vi "INS_civitanavi_write_PXI_subvi.vi"(4 "Send":bool, 8 "NavOn":bool, 9 "Init":bool, 11 "Cluster":T1={"Offset Roll"=0.726926, "Offset Pitch"=-0.17842, "Offset Heading"=0.0310803, "Azimuth"=0.0, "Latitude "=-23.213156, "Longitude"=-45.860622, "Height"=622.367, "LP_Vel_Z-North"=0.0, "LP_Vel_Y-East"=0.0, "LP_Vel_X-Up"=0.0}) -> (3 "string out":string)   [LabVIEW 2017]
panel:
  in  "Fact Reserved":bool
  in  "Download":bool
  in  "Fact Config":bool
  out "Half Second":bool[][](array[boolean])=[[FALSE, FALSE, FALSE, FALSE, FALSE, FALSE, FALSE, FALSE, FALSE, FALSE], [FALSE, FALSE, TRUE, TRUE, TRUE, TRUE, TRUE, FALSE, FALSE, FALSE], [FALSE, TRUE, FALSE, FALSE, FALSE, FALSE, FALSE, TRUE, FALSE, FALSE], [FALSE, TRUE, FALSE, FALSE, FALSE, FALSE, FALSE, TRUE, FALSE, FALSE], [FALSE, TRUE, FALSE, FALSE, FALSE, FALSE, FALSE, TRUE, FALSE, FALSE], [FALSE, TRUE, FALSE, FALSE, FALSE, FALSE, FALSE, TRUE, FALSE, FALSE], [FALSE, TRUE, FALSE, FALSE, FALSE, FALSE, FALSE, TRUE, FALSE, FALSE], [FALSE, TRUE, FALSE, FALSE, FALSE, FALSE, FALSE, TRUE, FALSE, FALSE], [FALSE, FALSE, TRUE, TRUE, TRUE, TRUE, TRUE, FALSE, FALSE, FALSE], [FALSE, FALSE, FALSE, FALSE, FALSE, FALSE, FALSE, FALSE, FALSE, FALSE]]
  out "Min 1":bool[][](array[boolean])=[[FALSE, FALSE, FALSE, FALSE, FALSE, FALSE, FALSE, FALSE, FALSE, FALSE], [FALSE, FALSE, TRUE, TRUE, TRUE, TRUE, TRUE, FALSE, FALSE, FALSE], [FALSE, TRUE, FALSE, FALSE, FALSE, FALSE, FALSE, TRUE, FALSE, FALSE], [FALSE, TRUE, FALSE, FALSE, FALSE, FALSE, FALSE, TRUE, FALSE, FALSE], [FALSE, TRUE, FALSE, FALSE, FALSE, FALSE, FALSE, TRUE, FALSE, FALSE], [FALSE, TRUE, FALSE, FALSE, FALSE, FALSE, FALSE, TRUE, FALSE, FALSE], [FALSE, TRUE, FALSE, FALSE, FALSE, FALSE, FALSE, TRUE, FALSE, FALSE], [FALSE, TRUE, FALSE, FALSE, FALSE, FALSE, FALSE, TRUE, FALSE, FALSE], [FALSE, FALSE, TRUE, TRUE, TRUE, TRUE, TRUE, FALSE, FALSE, FALSE], [FALSE, FALSE, FALSE, FALSE, FALSE, FALSE, FALSE, FALSE, FALSE, FALSE]]
  out "Min 0":bool[][](array[boolean])=[[FALSE, FALSE, FALSE, FALSE, FALSE, FALSE, FALSE, FALSE, FALSE, FALSE], [FALSE, FALSE, TRUE, TRUE, TRUE, TRUE, TRUE, FALSE, FALSE, FALSE], [FALSE, TRUE, FALSE, FALSE, FALSE, FALSE, FALSE, TRUE, FALSE, FALSE], [FALSE, TRUE, FALSE, FALSE, FALSE, FALSE, FALSE, TRUE, FALSE, FALSE], [FALSE, TRUE, FALSE, FALSE, FALSE, FALSE, FALSE, TRUE, FALSE, FALSE], [FALSE, TRUE, FALSE, FALSE, FALSE, FALSE, FALSE, TRUE, FALSE, FALSE], [FALSE, TRUE, FALSE, FALSE, FALSE, FALSE, FALSE, TRUE, FALSE, FALSE], [FALSE, TRUE, FALSE, FALSE, FALSE, FALSE, FALSE, TRUE, FALSE, FALSE], [FALSE, FALSE, TRUE, TRUE, TRUE, TRUE, TRUE, FALSE, FALSE, FALSE], [FALSE, FALSE, FALSE, FALSE, FALSE, FALSE, FALSE, FALSE, FALSE, FALSE]]
  out "Hour 1":bool[][](array[boolean])=[[FALSE, FALSE, FALSE, FALSE, FALSE, FALSE, FALSE, FALSE, FALSE, FALSE], [FALSE, FALSE, TRUE, TRUE, TRUE, TRUE, TRUE, FALSE, FALSE, FALSE], [FALSE, TRUE, FALSE, FALSE, FALSE, FALSE, FALSE, TRUE, FALSE, FALSE], [FALSE, TRUE, FALSE, FALSE, FALSE, FALSE, FALSE, TRUE, FALSE, FALSE], [FALSE, TRUE, FALSE, FALSE, FALSE, FALSE, FALSE, TRUE, FALSE, FALSE], [FALSE, TRUE, FALSE, FALSE, FALSE, FALSE, FALSE, TRUE, FALSE, FALSE], [FALSE, TRUE, FALSE, FALSE, FALSE, FALSE, FALSE, TRUE, FALSE, FALSE], [FALSE, TRUE, FALSE, FALSE, FALSE, FALSE, FALSE, TRUE, FALSE, FALSE], [FALSE, FALSE, TRUE, TRUE, TRUE, TRUE, TRUE, FALSE, FALSE, FALSE], [FALSE, FALSE, FALSE, FALSE, FALSE, FALSE, FALSE, FALSE, FALSE, FALSE]]
  out "Hour 0":bool[][](array[boolean])=[[FALSE, FALSE, FALSE, FALSE, FALSE, FALSE, FALSE, FALSE, FALSE, FALSE], [FALSE, FALSE, TRUE, TRUE, TRUE, TRUE, TRUE, FALSE, FALSE, FALSE], [FALSE, TRUE, FALSE, FALSE, FALSE, FALSE, FALSE, TRUE, FALSE, FALSE], [FALSE, TRUE, FALSE, FALSE, FALSE, FALSE, FALSE, TRUE, FALSE, FALSE], [FALSE, TRUE, FALSE, FALSE, FALSE, FALSE, FALSE, TRUE, FALSE, FALSE], [FALSE, TRUE, FALSE, FALSE, FALSE, FALSE, FALSE, TRUE, FALSE, FALSE], [FALSE, TRUE, FALSE, FALSE, FALSE, FALSE, FALSE, TRUE, FALSE, FALSE], [FALSE, TRUE, FALSE, FALSE, FALSE, FALSE, FALSE, TRUE, FALSE, FALSE], [FALSE, FALSE, TRUE, TRUE, TRUE, TRUE, TRUE, FALSE, FALSE, FALSE], [FALSE, FALSE, FALSE, FALSE, FALSE, FALSE, FALSE, FALSE, FALSE, FALSE]]
  out "string in":string
  out "DV_Word":bool[](array[boolean])
  out "B_55":u8 format="%x"
  out "B_54":u8 format="%x"
  out "String":string
  # "B#55 (Configuration and Command Mode)"
  # "0x35"
  # "roll 0.229593"
  # "0xBD"
  # "pitch 0.442368"
  # "0XFA"
  # "yaw 0.00104293"
  # "0XEE"
  # "0XAB"
  # "0.128098 LP_Y-East"
  # "Não deixar os botões selecionados"
  # "0.467339 LP_Z-North"
  # "B#54 (Data Validity Word)"
  # "1= Installation Offset input valid data\n1= Launch Azimuth geodetic orientation, position, (lat, long, height) valid \n1= Velocity input valid data \nRFU\nRFU\nRFU\n 7,6     00= \"Init Cmd\" (Configuration parameters setting)\n           10= \"NAV_On\"\n           01= Reserved\n           11= Enter Configuration Mode"
  # "0\n1\n2\n3\n4\n5\n6\n7"
  # "Atualizar os valores das variaveis e pulsar o botão send"
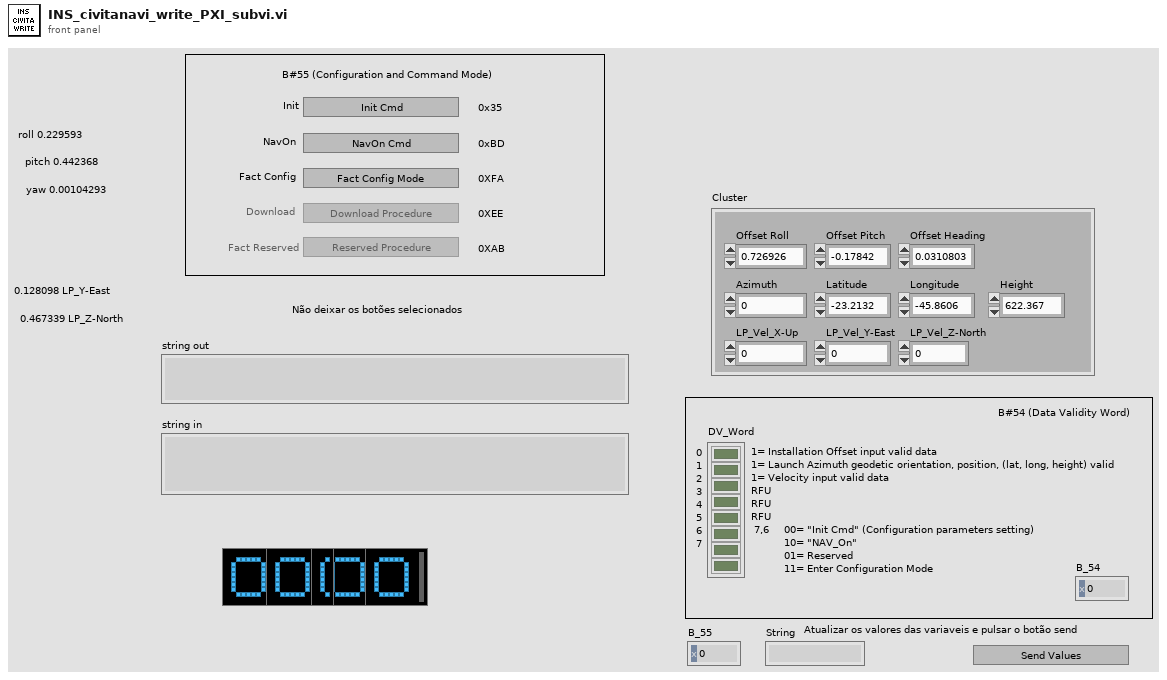
[diagram p1: front panel]
types:
  T1 = cluster{"Offset Roll":sgl, "Offset Pitch":sgl, "Offset Heading":sgl, "Azimuth":sgl, "Latitude ":sgl, "Longitude":sgl, "Height":sgl, "LP_Vel_Z-North":sgl, "LP_Vel_Y-East":sgl, "LP_Vel_X-Up":sgl}
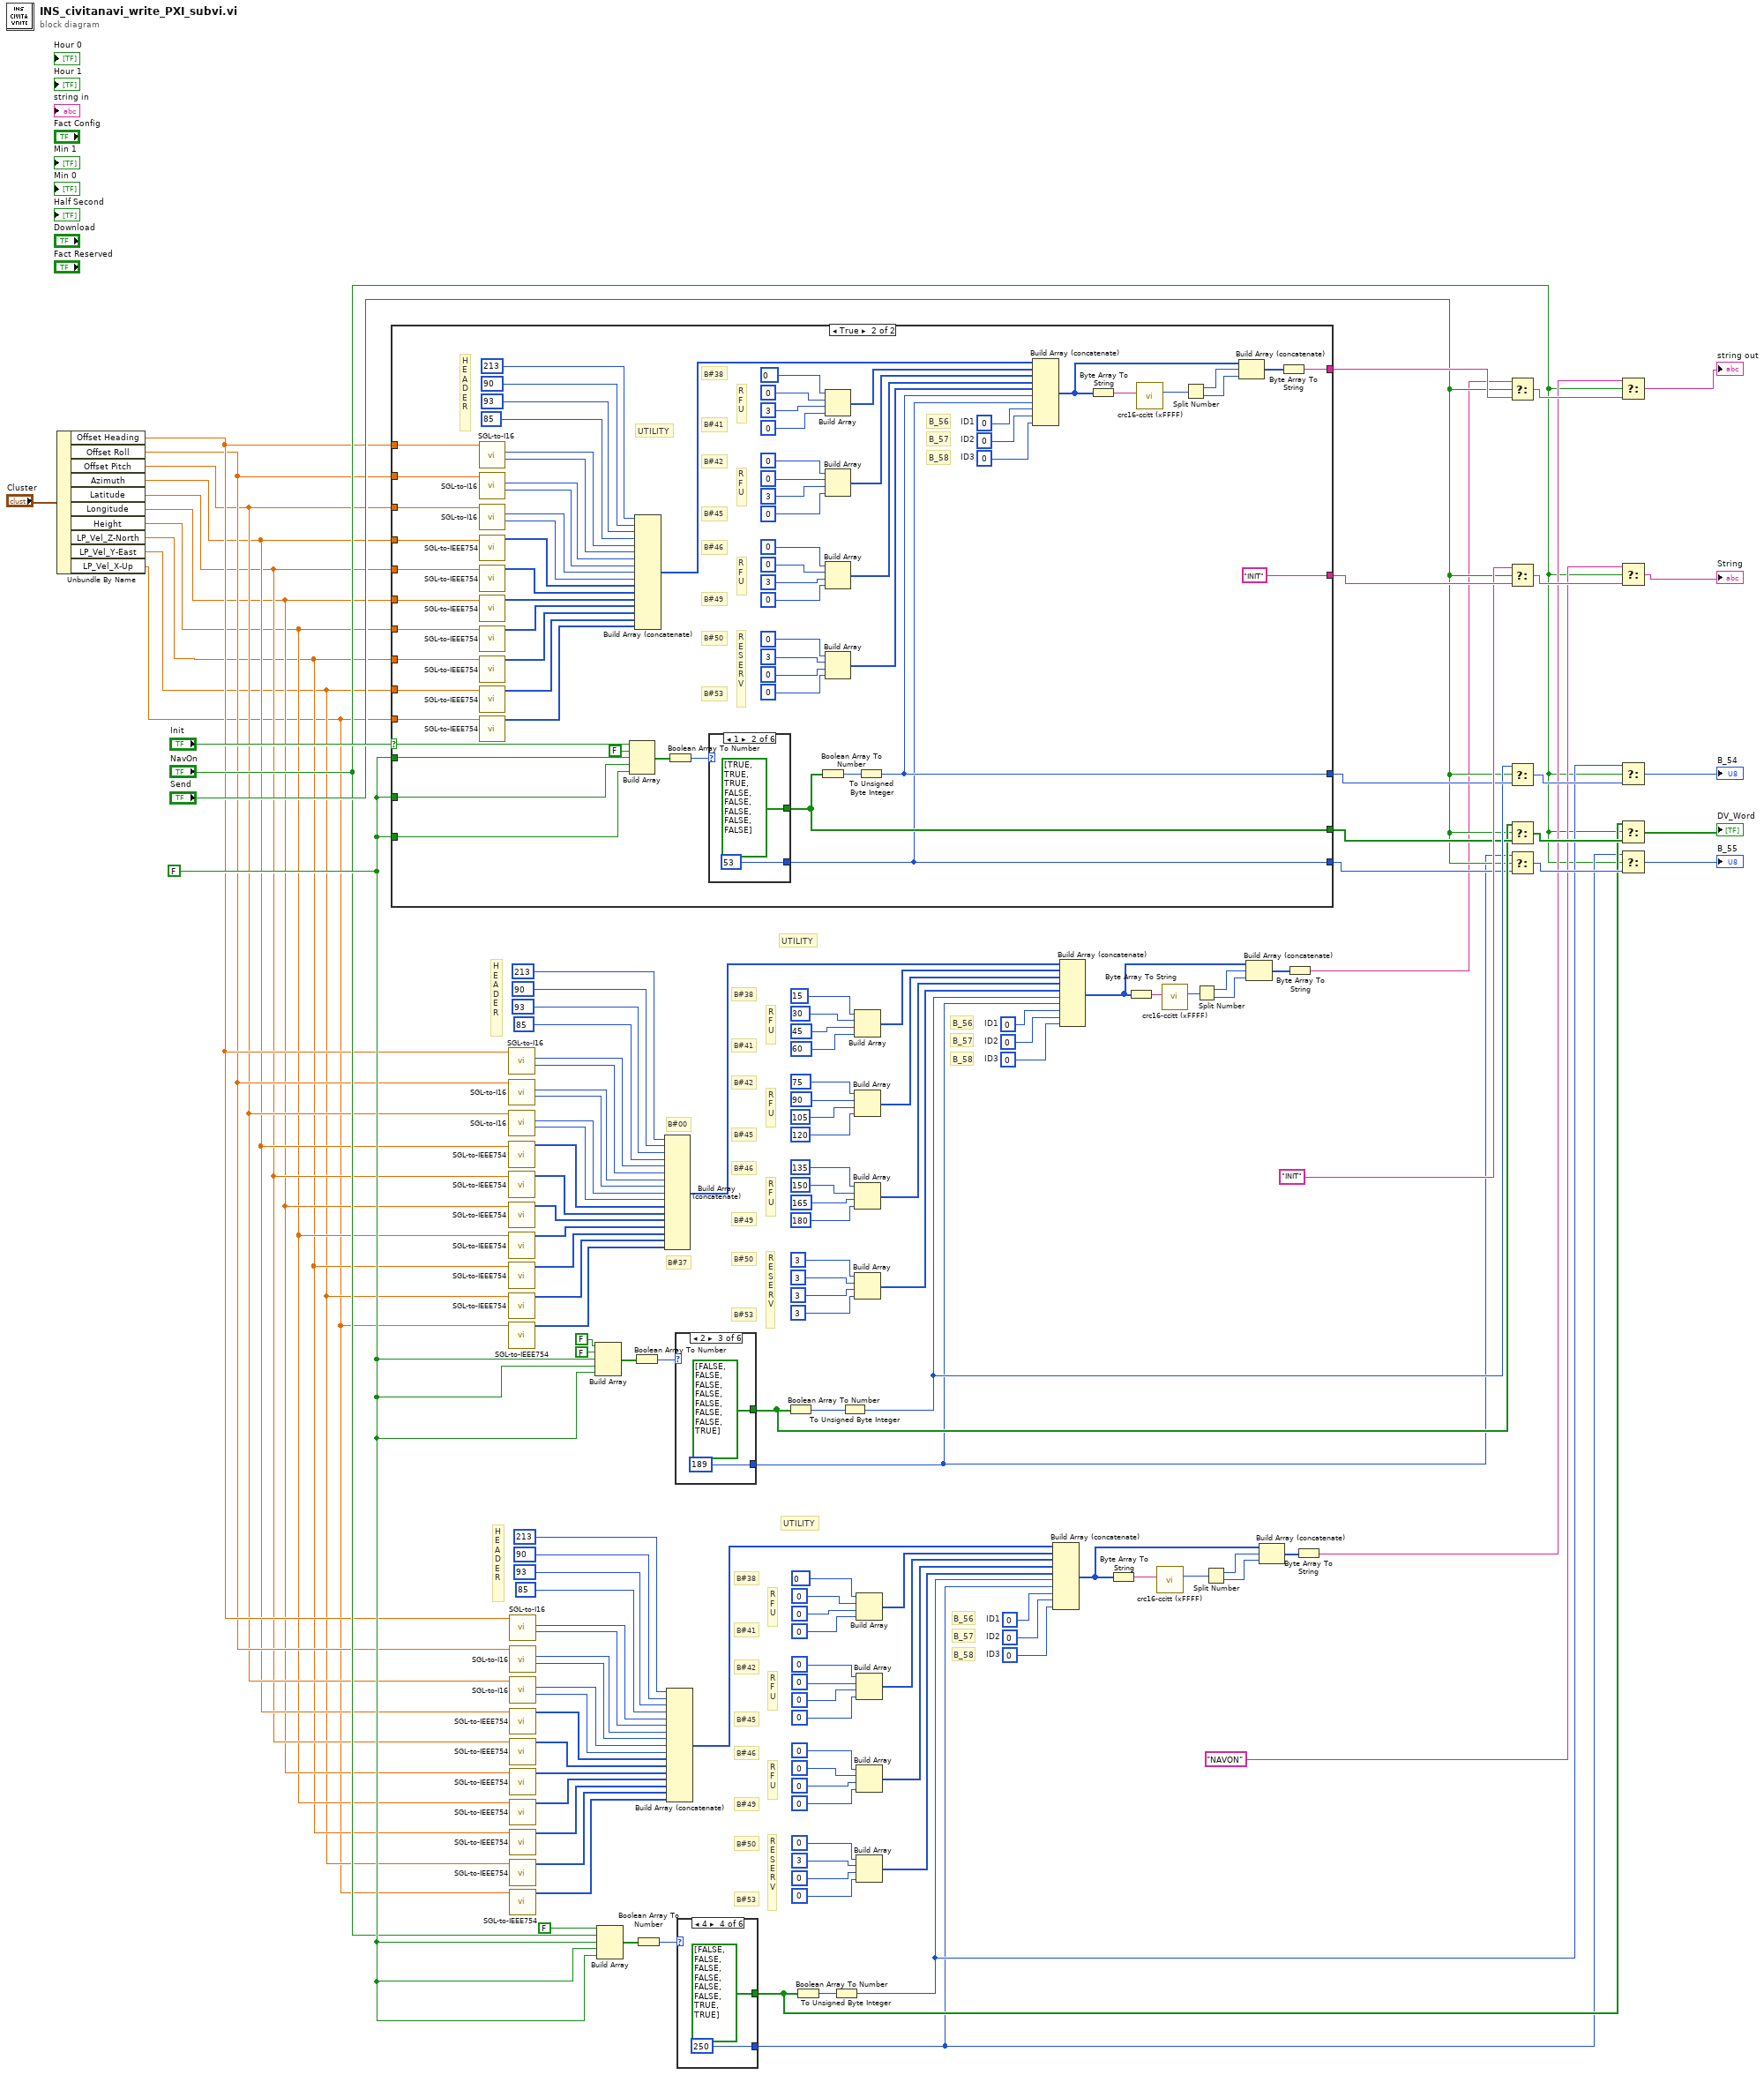
[diagram p0: block diagram]
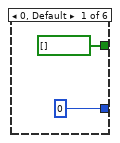
[diagram p2: hidden frame]
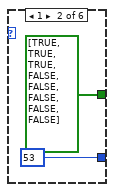
[diagram p3: hidden frame]
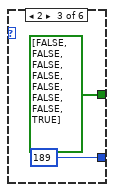
[diagram p4: hidden frame]
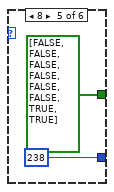
[diagram p5: hidden frame]
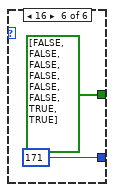
[diagram p6: hidden frame]
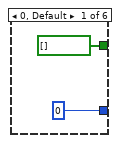
[diagram p7: hidden frame]
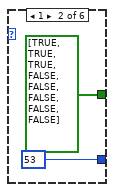
[diagram p8: hidden frame]
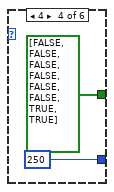
[diagram p9: hidden frame]
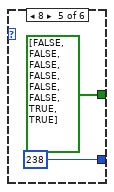
[diagram p10: hidden frame]
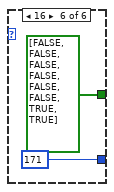
[diagram p11: hidden frame]
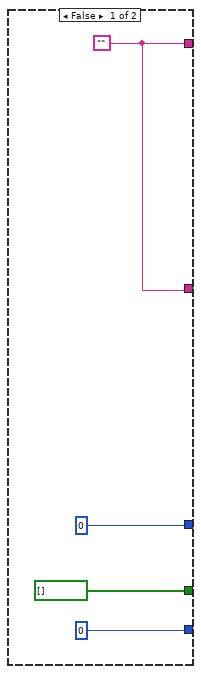
[diagram p12: hidden frame]
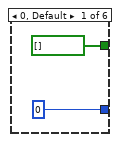
[diagram p13: hidden frame]
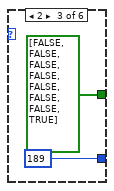
[diagram p14: hidden frame]
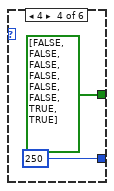
[diagram p15: hidden frame]
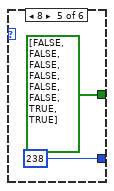
[diagram p16: hidden frame]
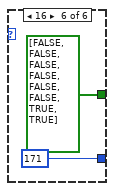
[diagram p17: hidden frame]
diagram:
  w63 = u8 0  # ID3
  w62 = u8 0  # ID2
  w61 = u8 0  # ID1
  w134 = u8 0  # ID3
  w133 = u8 0  # ID2
  w132 = u8 0  # ID1
  w19 = FALSE ("element")
  # "B#53"
  # "B#50"
  # "B#49"
  # "B#46"
  # "B#45"
  # "B#42"
  # "B#41"
  # "B#38"
  # "B_58"
  # "B_57"
  # "B_56"
  # "R\nE\nS\nE\nR\nV"
  # "R\nF\nU"
  # "R\nF\nU"
  # "R\nF\nU"
  # "H\nE\nA\nD\nE\nR"
  # "UTILITY"
  # "B#53"
  # "B#50"
  # "B#49"
  # "B#46"
  # "B#45"
  # "B#42"
  # "B#41"
  # "B#38"
  # "B#37"
  # "B#00"
  # "B_58"
  # "B_57"
  # "B_56"
  # "R\nE\nS\nE\nR\nV"
  # "R\nF\nU"
  # "R\nF\nU"
  # "R\nF\nU"
  # "H\nE\nA\nD\nE\nR"
  # "UTILITY"
  n1 = Unbundle By Name("Cluster") -> ("Offset Heading"=w11:sgl, "Offset Roll"=w10:sgl, "Offset Pitch"=w9:sgl, "Azimuth"=w8:sgl, "Latitude"=w7:sgl, "Longitude"=w6:sgl, "Height"=w5:sgl, "LP_Vel_Z-North"=w4:sgl, "LP_Vel_Y-East"=w3:sgl, "LP_Vel_X-Up"=w2:sgl)
  n2 = case shown="True" "Init" {
    selector: "Init" -> [_ w163]
    tunnel: w19 -> [_ w166]
    tunnel: w19 -> [_ w165]
    tunnel: w19 -> [_ w164]
    tunnel: w11 -> [_ w162]
    tunnel: w10 -> [_ w161]
    tunnel: w9 -> [_ w160]
    tunnel: w8 -> [_ w159]
    tunnel: w7 -> [_ w158]
    tunnel: w6 -> [_ w157]
    tunnel: w5 -> [_ w156]
    tunnel: w4 -> [_ w155]
    tunnel: w3 -> [_ w154]
    tunnel: w2 -> [_ w153]
    tunnel: [w144 "INIT"] -> w89
    tunnel: [w144 w151] -> w90
    tunnel: [u8 0 w150] -> w87
    tunnel: [bool[] [] ("DV_Word") w149] -> w85
    tunnel: [u8 0 w148] -> w83
    frame False {
      w144 = ""
    }
    frame True {
      w210 = u8 0  # ID3
      w209 = u8 0  # ID2
      w208 = u8 0  # ID1
      # "B#53"
      # "B#50"
      # "B#49"
      # "B#46"
      # "B#45"
      # "B#42"
      # "B#41"
      # "B#38"
      # "B_58"
      # "B_57"
      # "B_56"
      # "R\nE\nS\nE\nR\nV"
      # "R\nF\nU"
      # "R\nF\nU"
      # "R\nF\nU"
      # "H\nE\nA\nD\nE\nR"
      # "UTILITY"
      n3 = call "SGL-to-I16.vi"("Range"=w162) -> ("lo(x)"=w175:u8, "hi(x)"=w174:u8)  [unwired: 8 in, 1 out]
      n4 = call "SGL-to-I16.vi"("Range"=w161) -> ("lo(x)"=w177:u8, "hi(x)"=w176:u8)  [unwired: 8 in, 1 out]
      n5 = call "SGL-to-I16.vi"("Range"=w160) -> ("lo(x)"=w179:u8, "hi(x)"=w178:u8)  [unwired: 8 in, 1 out]
      n6 = call "SGL-to-IEEE754.vi"("Input_DBL"=w159) -> ("Output_U8"=w180:u8[])  [unwired: 10 in]
      n7 = call "SGL-to-IEEE754.vi"("Input_DBL"=w158) -> ("Output_U8"=w181:u8[])  [unwired: 10 in]
      n8 = call "SGL-to-IEEE754.vi"("Input_DBL"=w157) -> ("Output_U8"=w182:u8[])  [unwired: 10 in]
      n9 = call "SGL-to-IEEE754.vi"("Input_DBL"=w156) -> ("Output_U8"=w183:u8[])  [unwired: 10 in]
      n10 = call "SGL-to-IEEE754.vi"("Input_DBL"=w155) -> ("Output_U8"=w184:u8[])  [unwired: 10 in]
      n11 = call "SGL-to-IEEE754.vi"("Input_DBL"=w154) -> ("Output_U8"=w185:u8[])  [unwired: 10 in]
      n12 = call "SGL-to-IEEE754.vi"("Input_DBL"=w153) -> ("Output_U8"=w186:u8[])  [unwired: 10 in]
      n13 = Build Array(w163, FALSE ("element"), w166, w165, w164) -> (w168:bool[])
      n14 = Build Array (concatenate)(u8 213, u8 90, u8 93, u8 85, w174, w175, w176, w177, w178, w179, w180, w181, w182, w183, w184, w185, w186) -> (w203:u8[])
      n15 = Boolean Array To Number(Boolean array=w168) -> (number=w169:u32)
      n16 = case shown="1" w169 {
        tunnel: [u8 0 u8 53 u8 189 u8 250 u8 238 u8 171] -> w148
        tunnel: [bool[] [] ("DV_Word") bool[] [TRUE, TRUE, TRUE, FALSE, FALSE, FALSE, FALSE, FALSE] ("DV_Word") bool[] [FALSE, FALSE, FALSE, FALSE, FALSE, FALSE, FALSE, TRUE] ("DV_Word") bool[] [FALSE, FALSE, FALSE, FALSE, FALSE, FALSE, TRUE, TRUE] ("DV_Word") bool[] [FALSE, FALSE, FALSE, FALSE, FALSE, FALSE, TRUE, TRUE] ("DV_Word") bool[] [FALSE, FALSE, FALSE, FALSE, FALSE, FALSE, TRUE, TRUE] ("DV_Word")] -> w149
        frame 0, Default {
        }
        frame 1 {
        }
        frame 2 {
        }
        frame 4 {
        }
        frame 8 {
        }
        frame 16 {
        }
      }
      n17 = Boolean Array To Number(Boolean array=w149) -> (number=w167:u32)
      n18 = Build Array(u8 0, u8 0, u8 3, u8 0) -> (w204:u8[])
      n19 = Build Array(u8 0, u8 0, u8 3, u8 0) -> (w205:u8[])
      n20 = Build Array(u8 0, u8 0, u8 3, u8 0) -> (w206:u8[])
      n21 = Build Array(u8 0, u8 3, u8 0, u8 0) -> (w207:u8[])
      n22 = To Unsigned Byte Integer(number=w167) -> (unsigned 8bit integer=w150:u8)
      n23 = Build Array (concatenate)(w203, w204, w205, w206, w207, w150, w148, w208, w209, w210) -> (w213:u8[])
      n24 = Byte Array To String(unsigned byte array=w213) -> (string=w211:string)
      n25 = call "crc16-ccitt (xFFFF).vi"("Message"=w211) -> ("CRC"=w212:u16)  [unwired: 9 in, 1 out]
      n26 = Split Number(x=w212) -> (hi(x)=w214:u8, lo(x)=w215:u8)
      n27 = Build Array (concatenate)(w213, w214, w215) -> (w216:u8[])
      n28 = Byte Array To String(unsigned byte array=w216) -> (string=w151:string)
    }
  }
  n29 = call "SGL-to-I16.vi"("Range"=w11) -> ("lo(x)"=w99:u8, "hi(x)"=w98:u8)  [unwired: 8 in, 1 out]
  n30 = call "SGL-to-I16.vi"("Range"=w10) -> ("lo(x)"=w101:u8, "hi(x)"=w100:u8)  [unwired: 8 in, 1 out]
  n31 = call "SGL-to-I16.vi"("Range"=w9) -> ("lo(x)"=w103:u8, "hi(x)"=w102:u8)  [unwired: 8 in, 1 out]
  n32 = call "SGL-to-IEEE754.vi"("Input_DBL"=w8) -> ("Output_U8"=w104:u8[])  [unwired: 10 in]
  n33 = call "SGL-to-IEEE754.vi"("Input_DBL"=w7) -> ("Output_U8"=w105:u8[])  [unwired: 10 in]
  n34 = call "SGL-to-IEEE754.vi"("Input_DBL"=w6) -> ("Output_U8"=w106:u8[])  [unwired: 10 in]
  n35 = call "SGL-to-IEEE754.vi"("Input_DBL"=w5) -> ("Output_U8"=w107:u8[])  [unwired: 10 in]
  n36 = call "SGL-to-IEEE754.vi"("Input_DBL"=w4) -> ("Output_U8"=w108:u8[])  [unwired: 10 in]
  n37 = call "SGL-to-IEEE754.vi"("Input_DBL"=w3) -> ("Output_U8"=w109:u8[])  [unwired: 10 in]
  n38 = call "SGL-to-IEEE754.vi"("Input_DBL"=w2) -> ("Output_U8"=w110:u8[])  [unwired: 10 in]
  n39 = call "SGL-to-I16.vi"("Range"=w11) -> ("lo(x)"=w28:u8, "hi(x)"=w27:u8)  [unwired: 8 in, 1 out]
  n40 = call "SGL-to-I16.vi"("Range"=w10) -> ("lo(x)"=w30:u8, "hi(x)"=w29:u8)  [unwired: 8 in, 1 out]
  n41 = call "SGL-to-I16.vi"("Range"=w9) -> ("lo(x)"=w32:u8, "hi(x)"=w31:u8)  [unwired: 8 in, 1 out]
  n42 = call "SGL-to-IEEE754.vi"("Input_DBL"=w8) -> ("Output_U8"=w33:u8[])  [unwired: 10 in]
  n43 = call "SGL-to-IEEE754.vi"("Input_DBL"=w7) -> ("Output_U8"=w34:u8[])  [unwired: 10 in]
  n44 = call "SGL-to-IEEE754.vi"("Input_DBL"=w6) -> ("Output_U8"=w35:u8[])  [unwired: 10 in]
  n45 = call "SGL-to-IEEE754.vi"("Input_DBL"=w5) -> ("Output_U8"=w36:u8[])  [unwired: 10 in]
  n46 = call "SGL-to-IEEE754.vi"("Input_DBL"=w4) -> ("Output_U8"=w37:u8[])  [unwired: 10 in]
  n47 = call "SGL-to-IEEE754.vi"("Input_DBL"=w3) -> ("Output_U8"=w38:u8[])  [unwired: 10 in]
  n48 = call "SGL-to-IEEE754.vi"("Input_DBL"=w2) -> ("Output_U8"=w39:u8[])  [unwired: 10 in]
  n49 = Build Array(FALSE ("element"), FALSE ("element"), w19, w19, w19) -> (w92:bool[])
  n50 = Build Array(FALSE ("element"), "NavOn", w19, w19, w19) -> (w21:bool[])
  n51 = Boolean Array To Number(Boolean array=w92) -> (number=w93:u32)
  n52 = Boolean Array To Number(Boolean array=w21) -> (number=w22:u32)
  n53 = Build Array (concatenate)(u8 213, u8 90, u8 93, u8 85, w98, w99, w100, w101, w102, w103, w104, w105, w106, w107, w108, w109, w110) -> (w127:u8[])
  n54 = Build Array (concatenate)(u8 213, u8 90, u8 93, u8 85, w27, w28, w29, w30, w31, w32, w33, w34, w35, w36, w37, w38, w39) -> (w56:u8[])
  n55 = case shown="2" w93 {
    tunnel: [u8 0 u8 53 u8 189 u8 250 u8 238 u8 171] -> w81
    tunnel: [bool[] [] ("DV_Word") bool[] [TRUE, TRUE, TRUE, FALSE, FALSE, FALSE, FALSE, FALSE] ("DV_Word") bool[] [FALSE, FALSE, FALSE, FALSE, FALSE, FALSE, FALSE, TRUE] ("DV_Word") bool[] [FALSE, FALSE, FALSE, FALSE, FALSE, FALSE, TRUE, TRUE] ("DV_Word") bool[] [FALSE, FALSE, FALSE, FALSE, FALSE, FALSE, TRUE, TRUE] ("DV_Word") bool[] [FALSE, FALSE, FALSE, FALSE, FALSE, FALSE, TRUE, TRUE] ("DV_Word")] -> w84
    frame 0, Default {
    }
    frame 1 {
    }
    frame 2 {
    }
    frame 4 {
    }
    frame 8 {
    }
    frame 16 {
    }
  }
  n56 = case shown="4" w22 {
    tunnel: [u8 0 u8 53 u8 189 u8 250 u8 238 u8 171] -> w14
    tunnel: [bool[] [] ("DV_Word") bool[] [TRUE, TRUE, TRUE, FALSE, FALSE, FALSE, FALSE, FALSE] ("DV_Word") bool[] [FALSE, FALSE, FALSE, FALSE, FALSE, FALSE, FALSE, TRUE] ("DV_Word") bool[] [FALSE, FALSE, FALSE, FALSE, FALSE, FALSE, TRUE, TRUE] ("DV_Word") bool[] [FALSE, FALSE, FALSE, FALSE, FALSE, FALSE, TRUE, TRUE] ("DV_Word") bool[] [FALSE, FALSE, FALSE, FALSE, FALSE, FALSE, TRUE, TRUE] ("DV_Word")] -> w15
    frame 0, Default {
    }
    frame 1 {
    }
    frame 2 {
    }
    frame 4 {
    }
    frame 8 {
    }
    frame 16 {
    }
  }
  n57 = Boolean Array To Number(Boolean array=w84) -> (number=w91:u32)
  n58 = Boolean Array To Number(Boolean array=w15) -> (number=w20:u32)
  n59 = To Unsigned Byte Integer(number=w20) -> (unsigned 8bit integer=w16:u8)
  n60 = To Unsigned Byte Integer(number=w91) -> (unsigned 8bit integer=w86:u8)
  n61 = Build Array(u8 15, u8 30, u8 45, u8 60) -> (w128:u8[])
  n62 = Build Array(u8 75, u8 90, u8 105, u8 120) -> (w129:u8[])
  n63 = Build Array(u8 135, u8 150, u8 165, u8 180) -> (w130:u8[])
  n64 = Build Array(u8 3, u8 3, u8 3, u8 3) -> (w131:u8[])
  n65 = Build Array(u8 0, u8 0, u8 0, u8 0) -> (w57:u8[])
  n66 = Build Array(u8 0, u8 0, u8 0, u8 0) -> (w58:u8[])
  n67 = Build Array(u8 0, u8 0, u8 0, u8 0) -> (w59:u8[])
  n68 = Build Array(u8 0, u8 3, u8 0, u8 0) -> (w60:u8[])
  n69 = Build Array (concatenate)(w56, w57, w58, w59, w60, w16, w14, w61, w62, w63) -> (w66:u8[])
  n70 = Build Array (concatenate)(w127, w128, w129, w130, w131, w86, w81, w132, w133, w134) -> (w137:u8[])
  n71 = Byte Array To String(unsigned byte array=w66) -> (string=w64:string)
  n72 = Byte Array To String(unsigned byte array=w137) -> (string=w135:string)
  n73 = call "crc16-ccitt (xFFFF).vi"("Message"=w64) -> ("CRC"=w65:u16)  [unwired: 9 in, 1 out]
  n74 = call "crc16-ccitt (xFFFF).vi"("Message"=w135) -> ("CRC"=w136:u16)  [unwired: 9 in, 1 out]
  n75 = Split Number(x=w136) -> (hi(x)=w138:u8, lo(x)=w139:u8)
  n76 = Split Number(x=w65) -> (hi(x)=w67:u8, lo(x)=w68:u8)
  n77 = Build Array (concatenate)(w137, w138, w139) -> (w140:u8[])
  n78 = Build Array (concatenate)(w66, w67, w68) -> (w69:u8[])
  n79 = Byte Array To String(unsigned byte array=w140) -> (string=w1:string)
  n80 = Byte Array To String(unsigned byte array=w69) -> (string=w18:string)
  n81 = Select(t=w1, s="Send", f=w90) -> (s? t:f=w79:string)
  n82 = Select(t="INIT", s="Send", f=w89) -> (s? t:f=w78:string)
  n83 = Select(t=w86, s="Send", f=w87) -> (s? t:f=w76:u8)
  n84 = Select(t=w84, s="Send", f=w85) -> (s? t:f=w74:bool[])
  n85 = Select(t=w81, s="Send", f=w83) -> (s? t:f=w72:u8)
  n86 = Select(t=w18, s="NavOn", f=w79) -> (s? t:f=→"string out":string)
  n87 = Select(t="NAVON", s="NavOn", f=w78) -> (s? t:f=→"String":string)
  n88 = Select(t=w16, s="NavOn", f=w76) -> (s? t:f=→"B_54":u8)
  n89 = Select(t=w15, s="NavOn", f=w74) -> (s? t:f=→"DV_Word":bool[])
  n90 = Select(t=w14, s="NavOn", f=w72) -> (s? t:f=→"B_55":u8)
